vi "Write Over.vi"(8 "error in (no error)":errorcluster, 10 "Over":bool, 11 "33-Update Trace Data in":refnum<class "33-Update Trace Data.lvclass">) -> (0 "error out":errorcluster, 3 "33-Update Trace Data out":refnum<class "33-Update Trace Data.lvclass">)   [LabVIEW 2020, in "SECS Scenarios.lvlib" / "33-Update Trace Data.lvclass"]
uses:
  33-Update Trace Data.lvclass
  33-Update Trace Data.lvclass/33-Update Trace Data.ctl
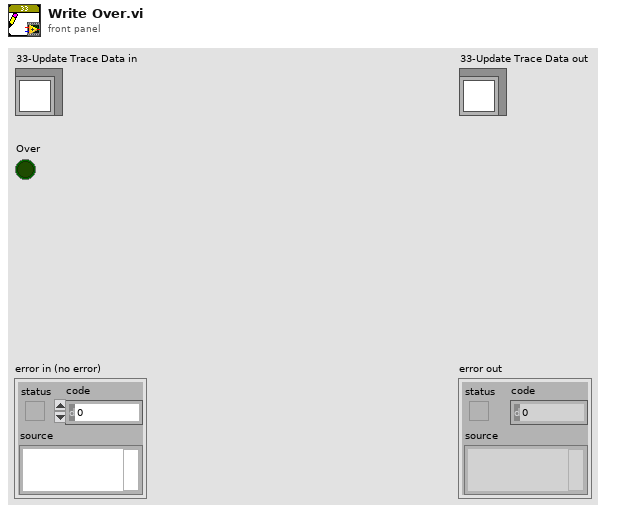
[diagram p1: front panel]
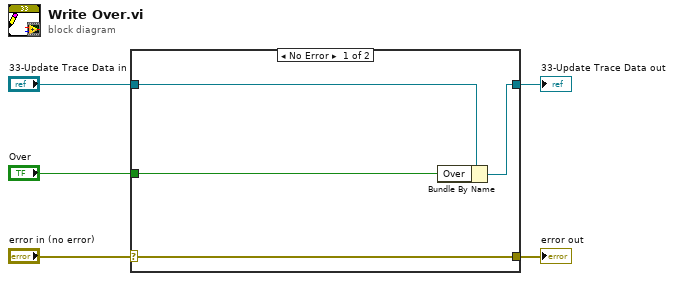
[diagram p0: block diagram]
diagram:
  n1 = case shown="No Error" "error in (no error)" {
    selector: "error in (no error)" -> [w9 w10]
    tunnel: [w9 w10] -> w4
    tunnel: [w7 w11] -> w2
    tunnel: "33-Update Trace Data in" -> [w8 w11]
    tunnel: "Over" -> [w6 _]
    frame No Error {
      n2 = Bundle By Name(cluster=w8, "Over"=w6) -> (w7:refnum<class "33-Update Trace Data.lvclass">)
    }
    frame Error {
    }
  }
  "error out" <- w4
  "33-Update Trace Data out" <- w2
